vi "myRIO_BRig_RT_dataCurrent_IallReward_L.vi"() -> (2 "output_IallReward_L":i32)   [LabVIEW 2014]
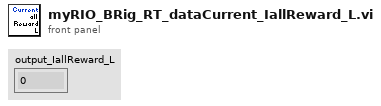
[diagram p1: front panel]
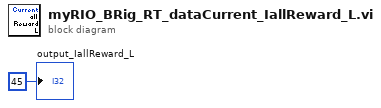
[diagram p0: block diagram]
diagram:
  "output_IallReward_L" <- 45 ("output_iBlock")
